vi "Write State.vi"(8 "error in (no error)":errorcluster, 10 "State":T1, 11 "Expansion in":refnum<class "Saturation.lvclass">) -> (0 "error out":errorcluster, 3 "Expansion out":refnum<class "Saturation.lvclass">)   [LabVIEW 2017, in "Saturation.lvclass"]
uses:
  Saturation.lvclass
  Type Defs/Saturation State.ctl
  Saturation.lvclass/Saturation.ctl
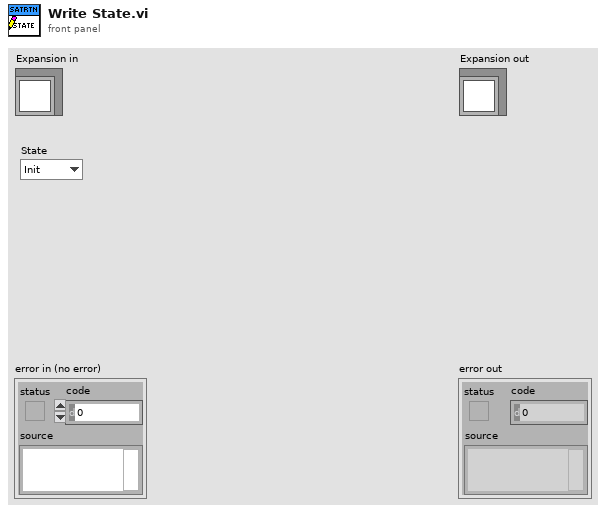
[diagram p1: front panel]
types:
  T1 = typedef "Saturation.lvclass/Saturation State.ctl" = enum16{"Init", "Update", "Go", "Control Valve", "Wait for Pressure", "Wait and Monitor", "Stop", "Idle", "Error", "Shutdown"}
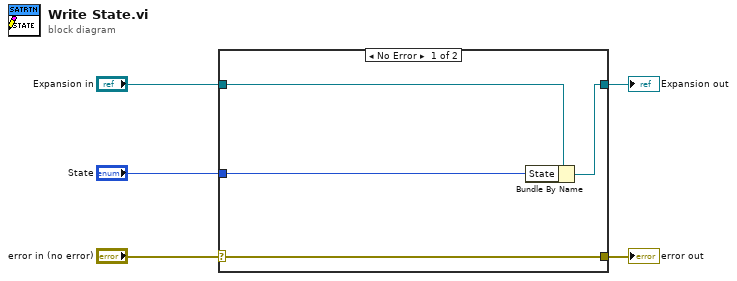
[diagram p0: block diagram]
diagram:
  n1 = case shown="No Error" "error in (no error)" {
    selector: "error in (no error)" -> [w9 w10]
    tunnel: [w9 w10] -> w4
    tunnel: [w7 w11] -> w2
    tunnel: "Expansion in" -> [w8 w11]
    tunnel: "State" -> [w6 _]
    frame No Error {
      n2 = Bundle By Name(cluster=w8, "State"=w6) -> (w7:refnum<class "Saturation.lvclass">)
    }
    frame Error {
    }
  }
  "error out" <- w4
  "Expansion out" <- w2
